vi "Motion control Custom motor.vi"(8 "error in (no error)":errorcluster, 11 "Datos de Nueva Adquisición":T1 {"Datos Osciloscopio"."Número Promedio" min=2 max=20; "Datos a Guardar In"."Posición Actual" format="%#_10f"; "Datos a Guardar In"."Posición Cero" format="%#_10f"; "Datos Bipolar/Unipolar"."Numero de lecturas" max=910098 step=1}) -> (0 "error out":errorcluster)   [LabVIEW 2017]
doc: "Mover los motores a pasos el numero d epasos seleccionados"
uses:
  Type Definitions/Asistente de adquisicion Cluster.ctl
  Type Definitions/Datos Zaber.ctl
  Type Definitions/parametros motores.ctl
  Type Definitions/Datos a Guardar.ctl
  Type Definitions/datos osciloscopio.ctl
  <instrlib>/Control de MaP/Public/Controls/Command to motor.ctl
  <vilib>/Platform/TimedLoop/XDataNode/timing_clust.ctl
  <vilib>/Platform/TimedLoop/XDataNode/nitl_modes.ctl
  <vilib>/Platform/TimedLoop/XDataNode/wakeup.ctl
  <vilib>/platform/TimedLoop/XDataNode/XDataNode.xnode
  <instrlib>/Control de MaP/Control de MaP.lvlib
  <vilib>/Platform/TimedLoop/XDataNode/XDNodeRunTimeDep.lvlib
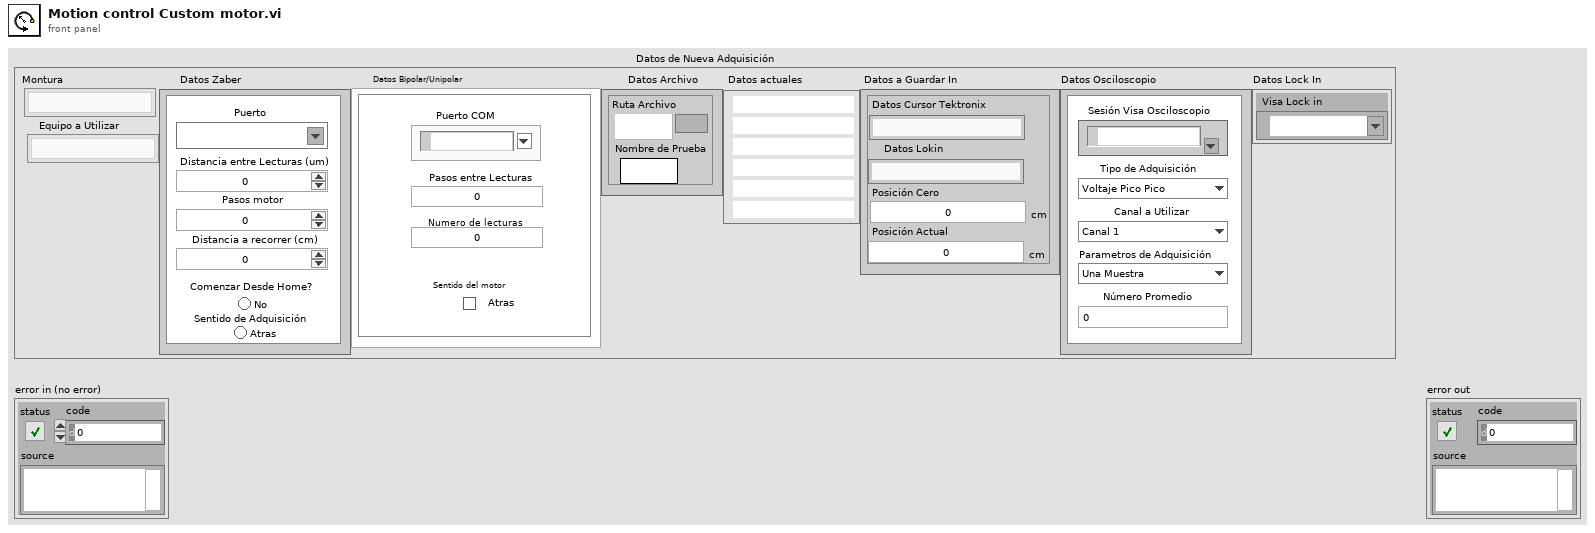
[diagram p1: front panel]
types:
  T1 = typedef "Asistente de adquisicion Cluster.ctl" = cluster{"Montura":enum16{"Zaber T-LSR450B", "Motor Bipolar", "Motor Unipolar"}, "Equipo a Utilizar":enum16{"SR830 Lock In", "TDS 2012B Osciloscope"}, "Datos Zaber":T2, "Datos Bipolar/Unipolar":T3, "Datos Archivo":cluster{"Ruta Archivo":path, "Nombre de Prueba":string}, "Datos actuales":cluster{"Montura":string, "Equipo":string, "Posición Actual":string, "Distancia Total a recorrer":string, "distancia Entre lecturas":string, "Pasos entre lecturas":string}, "Datos a Guardar In":T4, "Datos Osciloscopio":T5, "Datos Lock In":cluster{"Visa Lock in":refnum<visa-resource-name>}}
  T2 = typedef "Datos Zaber.ctl" = cluster{"Sentido de Adquisición":bool, "Comenzar Desde Home?":bool, "Distancia a recorrer (cm)":u32, "Pasos motor":i32, "Distancia entre Lecturas (um)":dbl, "Puerto":refnum<visa-resource-name>}
  T3 = typedef "parametros motores.ctl" = cluster{"Puerto COM":refnum<visa-resource-name>, "Pasos entre Lecturas":u16, "Numero de lecturas":u32, "Sentido del motor":bool}
  T4 = typedef "Datos a Guardar.ctl" = cluster{"Datos Cursor Tektronix":string, "Datos Lokin":string, "Posición Cero":dbl[unit], "Posición Actual":dbl[unit]}
  T5 = typedef "datos osciloscopio.ctl" = cluster{"Sesión Visa Osciloscopio":refnum<visa-resource-name>, "Tipo de Adquisición":enum16{"Voltaje Pico Pico", "Voltaje RMS", "Cursor Tiempo"}, "Canal a Utilizar":enum16{"Canal 1", "Canal 2", "Canal 1 y 2"}, "Parametros de Adquisición":enum16{"Una Muestra", "Promedio"}, "Número Promedio":i32}
  T6 = typedef "Control de MaP.lvlib/Command to motor.ctl" = cluster{"Dirección Bipolar":u8, "Dirección Unipolar":u8, "N°. Pasos Unipolar":u16, "N°. Pasos Bipolar":u16, "Velocidad":u8, "Tipo de paso":u8}
  T7 = typedef "XDNodeRunTimeDep.lvlib/timing_clust.ctl" = cluster{"Expected End [f-1]":u64, "Actual End [f-1]":u64, "Finished Late? [f-1]":bool, "Expected End [i-1]":u64, "Actual End [i-1]":u64, "Finished Late? [i-1]":bool, "Expected Start [i]":u64, "Actual Start [i]":u64, "Expected Start [f]":u64, "Actual Start [f]":u64, "Source Name":string, "Structure Name":string, "Period":i64, "Deadline":i64, "Offset":i64, "Start":i64, "Priority":i32, "Timeout":i32, "Mode":T8, "Wakeup Reason":T9, "Error":errorcluster, "Source Type":string, "Secondary Source Type":string, "Global End Time":u64, "Global Start Time":u64, "Frame Duration":u64, "Iteration Duration":u64, "Assigned CPU":i32, "I/O Scan Engine Mode":u32}
  T8 = typedef "XDNodeRunTimeDep.lvlib/nitl_modes.ctl" = enum32{"No Change", "Process missed periods, maintain original phase", "Discard missed periods, maintain original phase", "Process missed periods, ignore original phase", "Discard missed periods, ignore original phase"}
  T9 = typedef "XDNodeRunTimeDep.lvlib/wakeup.ctl" = enum32{"Normal", "Aborted", "Asynchronous wakeup", "Timing source error", "Timed loop error", "Timeout"}
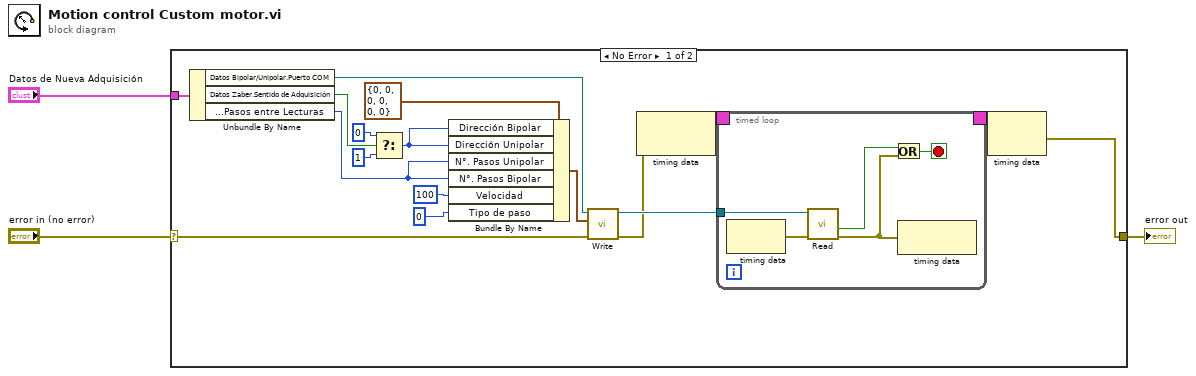
[diagram p0: block diagram]
diagram:
  n1 = case shown="No Error" "error in (no error)" {
    selector: "error in (no error)" -> [w16 w36]
    tunnel: "Datos de Nueva Adquisición" -> [w18 _]
    tunnel: [w5 w36] -> w2
    frame No Error {
      n2 = Unbundle By Name(w18) -> ("Datos Bipolar/Unipolar.Puerto COM"=w17:refnum<visa-resource-name>, "Datos Zaber.Sentido de Adquisición"=w15:bool, "Datos Bipolar/Unipolar.Pasos entre Lecturas"=w11:u16)
      n3 = Select(t=u8 0 ("Dirección Bipolar"), s=w15, f=u8 1) -> (s? t:f=w12:u8)
      n4 = Bundle By Name(cluster=T6 {"Dirección Bipolar"=0, "Dirección Unipolar"=0, "N°. Pasos Unipolar"=0, "N°. Pasos Bipolar"=0, "Velocidad"=0, "Tipo de paso"=0} ("Comando"), "Dirección Bipolar"=w12, "Dirección Unipolar"=w12, "N°. Pasos Unipolar"=w11, "N°. Pasos Bipolar"=w11, "Velocidad"=u8 100, "Tipo de paso"=u8 0) -> (w20:T6)
      n5 = call <instrlib>:"Write.vi"("error in (no error)"=w16, "Comando"=w20, "VISA resource name"=w17) -> ("error out"=w4:errorcluster, "VISA resource name out"=w6:refnum<visa-resource-name>)  [unwired: 6 in, 1 out]
      n6 = node-c288(w4) -> (w8:T7)
      n7 = timed-loop {
        timing: w8 -> [_]
        timing-out: [_] -> w7
        tunnel: w6 -> [w23]
        stop <- w25 stop-if-true
        n8 = node-c288() -> (w22:errorcluster)  [unwired: 1 in]
        n9 = call <instrlib>:"Read.vi"("error in (no error)"=w22, "VISA resource name"=w23) -> ("error out"=w21:errorcluster, "End"=w24:bool)  [unwired: 6 in, 2 out]
        n10 = Or(x=w24, y=w21) -> (x .or. y?=w25:bool)
        n11 = node-c288(w21) -> ()  [unwired: 1 out]
      }
      n12 = node-c288(w7) -> (w5:errorcluster)
    }
    frame Error {
    }
  }
  "error out" <- w2
